vi "getRunCardData.vi"(8 "error in (no error)":errorcluster, 9 "Jobno":string, 11 "RCName":string="¯M¯N®É¶¡") -> (0 "error out":errorcluster, 2 "data":string)   [LabVIEW 2012]
uses:
  <vilib>/addons/database/Connection.llb/DB Tools Open Connec (Path).vi
  <vilib>/addons/database/Connection.llb/Conn Execute.vi
  <vilib>/addons/database/Recordset.llb/Rec Fetch Integer Data (R).vi
  <vilib>/addons/database/Recordset.llb/Rec Destroy - Connection.vi
  <vilib>/addons/database/Recordset.llb/Rec Fetch String Data (R).vi
  <vilib>/addons/database/NI_Database_API.lvlib
panel:
  out "concatenated string 2":string
  out "concatenated string":string
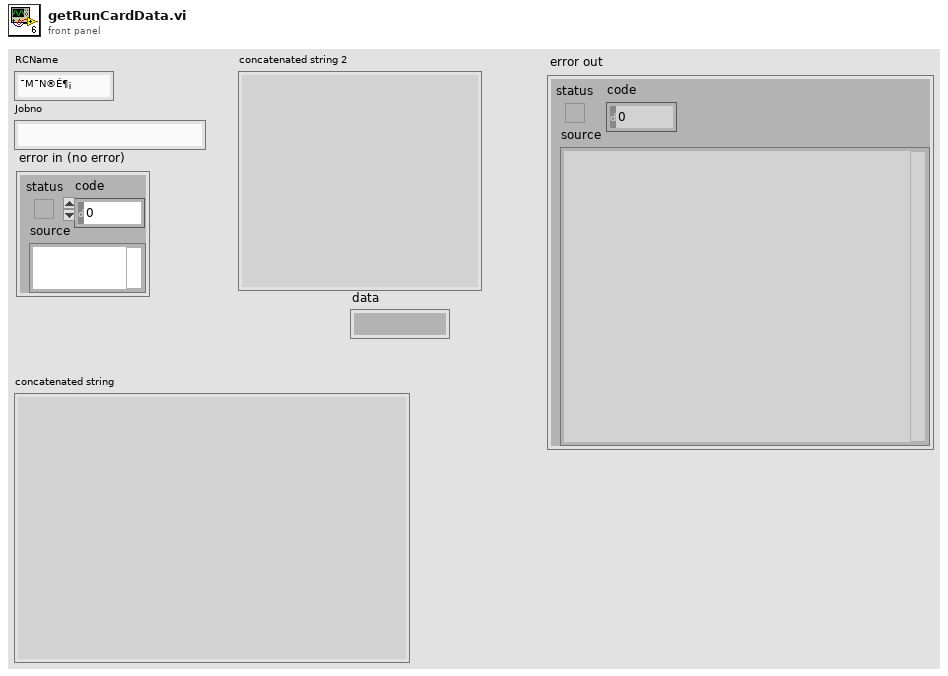
[diagram p1: front panel]
types:
  T1 = typedef "NI_Database_API.lvlib/Conn ObjectReference.ctl" = refnum<k1>
  T2 = typedef "NI_Database_API.lvlib/Rec ObjectReference.ctl" = refnum<k1>
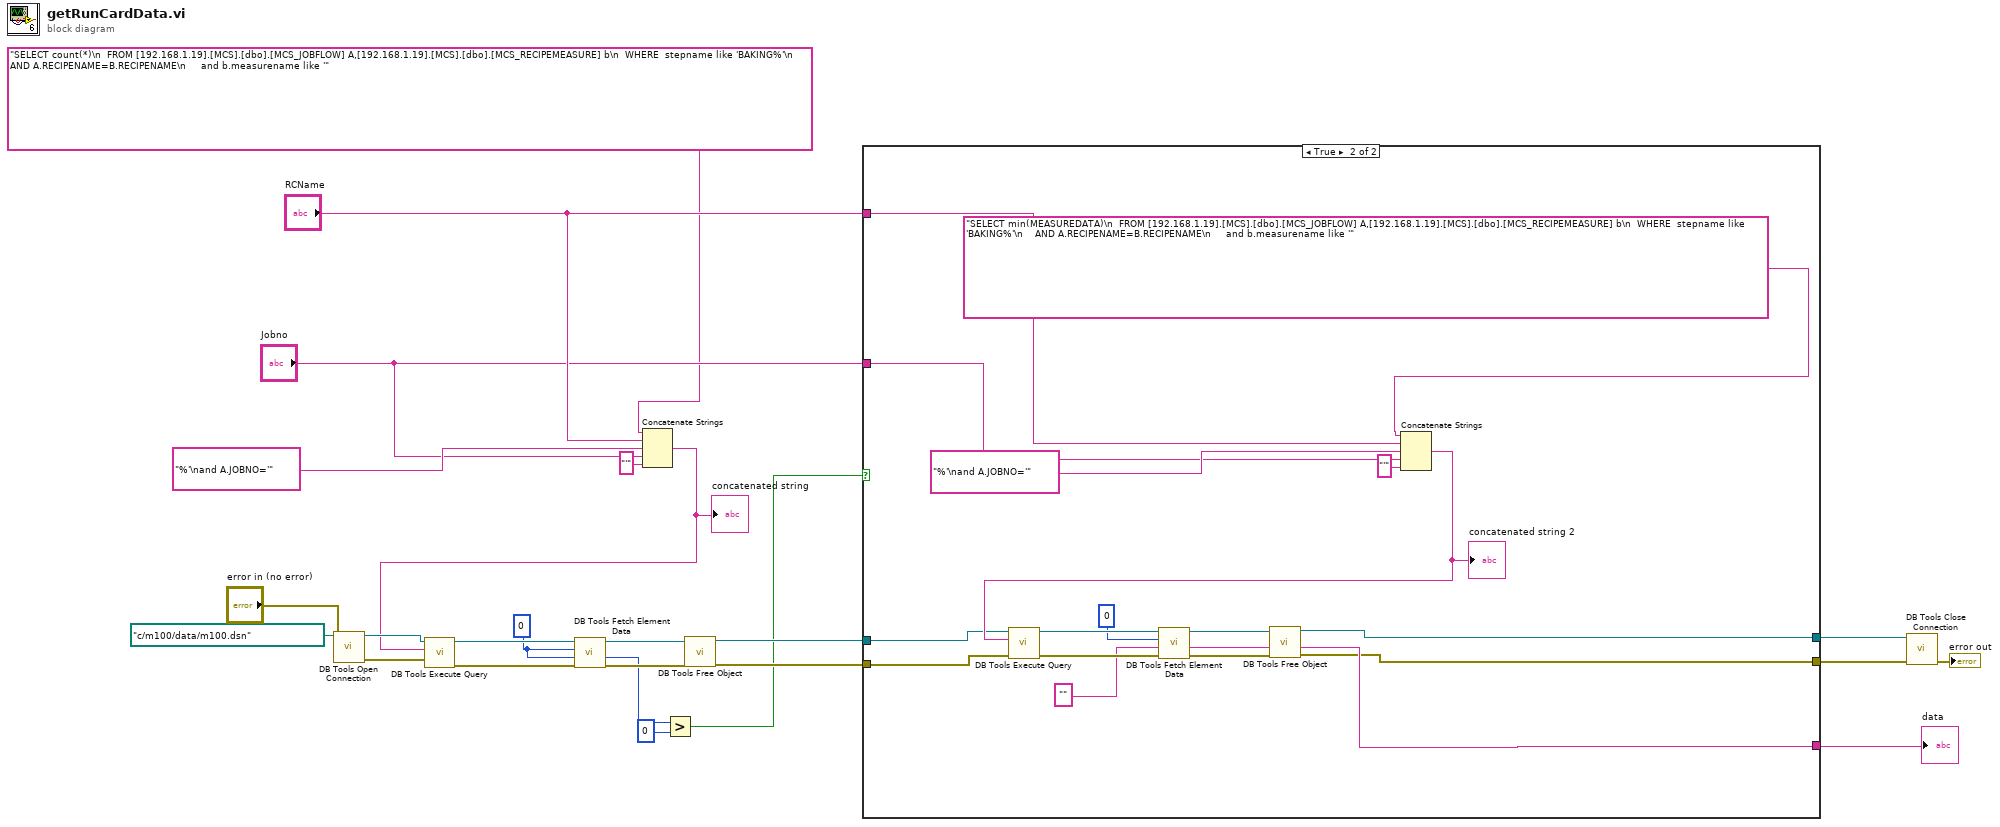
[diagram p0: block diagram]
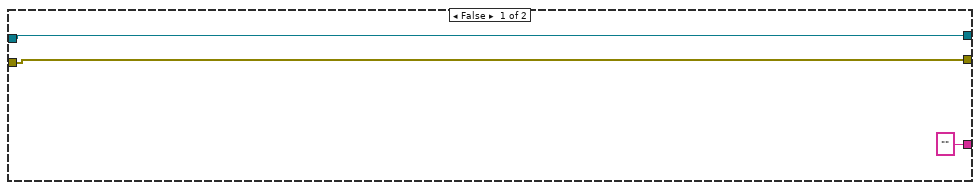
[diagram p2: hidden frame]
diagram:
  w16 = 0
  n1 = call-poly <vilib>:"DB Tools Open Connection.vi"("error in (no error)"="error in (no error)", "connection information"=path "c:/m100/data/m100.dsn") -> ("error out"=w17:errorcluster, "connection reference"=w18:T1)  [unwired: 6 in]
  n2 = Concatenate Strings("SELECT count(*)\n  FROM [192.168.1.19].[MCS].[dbo].[MCS_JOBFLOW] A,[192.168.1.19].[MCS].[dbo].[MCS_RECIPEMEASURE] b\n  WHERE  stepname like 'BAKING%'\n    AND A.RECIPENAME=B.RECIPENAME\n     and b.measurename like '", "RCName", "%'\nand A.JOBNO='" ("string"), "Jobno", "'" ("string")) -> (w10:string)
  "concatenated string" <- w10
  n3 = call-poly <vilib>:"DB Tools Execute Query.vi"("error in (no error)"=w17, "SQL query"=w10, "connection reference"=w18) -> ("error out"=w20:errorcluster, "recordset reference"=w22:T2)  [unwired: 5 in]
  n4 = call-poly <vilib>:"DB Tools Fetch Element Data.vi"("error in (no error)"=w20, "type"=w16, "column index"=w16, "recordset reference"=w22) -> ("error out"=w19:errorcluster, "data"=w9:i32, "recordset reference out"=w21:T2)  [unwired: 3 in]
  n5 = Greater?(x=w9, y=0) -> (0:w4:bool)
  n6 = call-poly <vilib>:"DB Tools Free Object.vi"("error in (no error)"=w19, "recordset reference"=w21) -> ("error out"=w5:errorcluster, "connection reference"=w6:T1)  [unwired: 8 in]
  n7 = case shown="True" w4 {
    tunnel: "RCName" -> [_ w35]
    tunnel: "Jobno" -> [_ w34]
    tunnel: ["" ("data") w32] -> w7
    tunnel: w6 -> [w26 w31]
    tunnel: w5 -> [w25 w30]
    tunnel: [w26 w29] -> w2
    tunnel: [w25 w28] -> w1
    frame False {
    }
    frame True {
      n8 = Concatenate Strings("SELECT min(MEASUREDATA)\n  FROM [192.168.1.19].[MCS].[dbo].[MCS_JOBFLOW] A,[192.168.1.19].[MCS].[dbo].[MCS_RECIPEMEASURE] b\n  WHERE  stepname like 'BAKING%'\n    AND A.RECIPENAME=B.RECIPENAME\n     and b.measurename like '", w35, "%'\nand A.JOBNO='" ("string"), w34, "'" ("string")) -> (w33:string)
      "concatenated string 2" <- w33
      n9 = call-poly <vilib>:"DB Tools Execute Query.vi"("error in (no error)"=w30, "SQL query"=w33, "connection reference"=w31) -> ("error out"=w42:errorcluster, "recordset reference"=w44:T2)  [unwired: 5 in]
      n10 = call-poly <vilib>:"DB Tools Fetch Element Data.vi"("error in (no error)"=w42, "type"="", "column index"=0, "recordset reference"=w44) -> ("error out"=w41:errorcluster, "data"=w32:string, "recordset reference out"=w43:T2)  [unwired: 3 in]
      n11 = call-poly <vilib>:"DB Tools Free Object.vi"("error in (no error)"=w41, "recordset reference"=w43) -> ("error out"=w28:errorcluster, "connection reference"=w29:T1)  [unwired: 8 in]
    }
  }
  "data" <- w7
  n12 = call <vilib>:"DB Tools Close Connection.vi"("error in (no error)"=w1, "connection reference"=w2) -> ("error out"=→"error out":errorcluster)  [unwired: 5 in]
